vi "LockinDAQ.Create.AO Task.vi"(8 "error in (no error)":errorcluster, 11 "LockinDAQ":refnum<class "LockinDAQ.lvclass">) -> (0 "error out":errorcluster, 3 "LockinDAQ out":refnum<class "LockinDAQ.lvclass">)   [LabVIEW 2016, in "LockinDAQ.lvclass"]
uses:
  LockinDAQ.lvclass
  LockinDAQ.lvclass/LockinDAQ.ctl
  <vilib>/DAQmx/create/channels.llb/DAQmx Create Channel (AO-Voltage-Basic).vi
  <resource>/objmgr/daqmx.rc
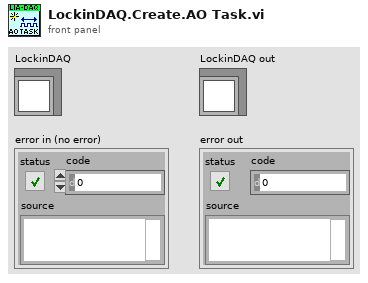
[diagram p1: front panel]
types:
  T1 = typedef "LockinDAQ.lvclass/AO.config-array.ctl" = T2[]
  T2 = typedef "LockinDAQ.lvclass/AO.config-cluster.ctl" = cluster{"AO.channels":tag, "AO.Range":T3, "output terminal configuration":i32, "DAQ Type":T4}
  T3 = typedef "LockinDAQ.lvclass/446xAO-enum.ctl" = enum16{"±0.1 V", "±1.0 V", "±10.0 V"}
  T4 = typedef "LockinDAQ.lvclass/DAQType-enum.ctl" = enum16{"None", "USB 4431", "PXI 446x"}
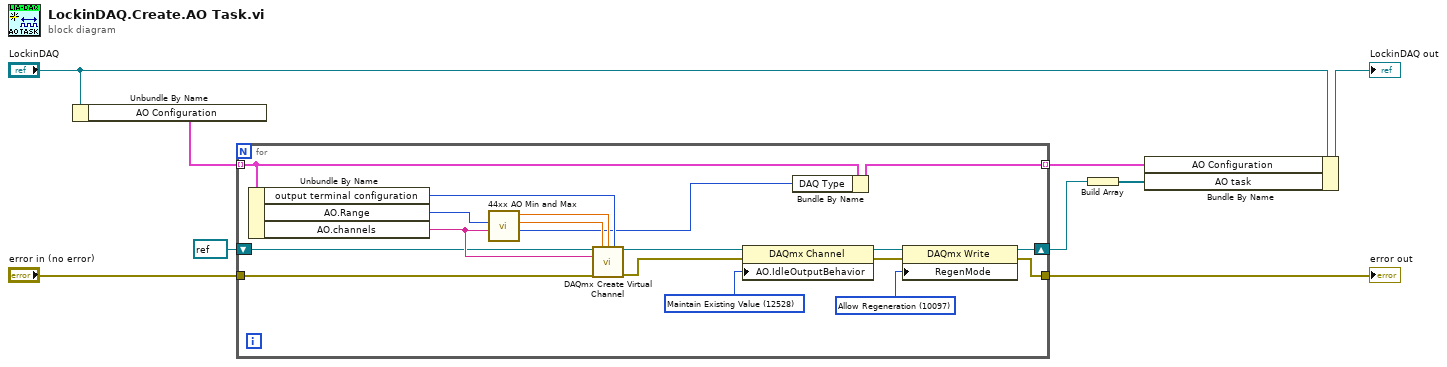
[diagram p0: block diagram]
diagram:
  n1 = Unbundle By Name("LockinDAQ") -> ("AO Configuration"=w8:T1)
  n2 = for {
    tunnel: "error in (no error)" -> [w24]
    tunnel: [w12] -> w6
    tunnel: w8 -> [w11] mode=indexing
    tunnel: [w16] -> w5 mode=indexing
    shift-right: [w18] -> w3
    shift-left: refnum<k21> refnum ("task out") -> [w10]
    w13 = 10097 items=["Allow Regeneration"=10097, "Do Not Allow Regeneration"=10158] ("RegenMode")
    w14 = 12528 items=["Zero Volts"=12526, "High-Impedance"=12527, "Maintain Existing Value"=12528] ("AO.IdleOutputBehavior")
    n3 = Unbundle By Name(w11) -> ("output terminal configuration"=w20:i32, "AO.Range"=w19:T3, "AO.channels"=w21:tag)
    n4 = call "44xx AO Min and Max.vi"("AO.channels"=w21, "AO.Range"=w19) -> ("DAQ Type"=w17:T4, "AO.max"=w23:dbl, "AO.min"=w22:dbl)  [unwired: 7 in]
    n5 = call-poly <vilib>:"DAQmx Create Virtual Channel.vi"("task in"=w10, "maximum value"=w23, "minimum value"=w22, "output terminal configuration"=w20, "physical channels"=w21, "error in"=w24) -> ("task out"=w27:refnum<k21>, "error out"=w15:errorcluster)  [unwired: 8 in]
    n6 = property class="DAQmx Channel"(reference=w27, error in=w15, "AO.IdleOutputBehavior"=w14) -> (reference out=w26:refnum<k21>, error out=w25:errorcluster)
    n7 = Bundle By Name(cluster=w11, "DAQ Type"=w17) -> (w16:T2)
    n8 = property class="DAQmx Write"(reference=w26, error in=w25, "RegenMode"=w13) -> (reference out=w18:refnum<k21>, error out=w12:errorcluster)
  }
  "error out" <- w6
  n9 = Build Array(w3) -> (w2:refnum<k21>[])
  n10 = Bundle By Name(cluster="LockinDAQ", "AO Configuration"=w5, "AO task"=w2) -> (→"LockinDAQ out":refnum<class "LockinDAQ.lvclass">)
